vi "Set Duty Cycle.vi"   [LabVIEW 2011, in "LMH-LINX.lvlib"]
doc: "Set the duty cycle of the specified PWM channel. \n\nA duty cycle of 0 coresponds to 0% on\nA duty cycle of .33 coresponds to 33% on\nA duty cycle of 1 coresponds to 100% on\netc"
uses:
  LMH-LINX.lvlib
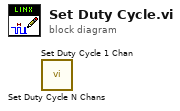
[diagram p0: block diagram]
diagram:
  n1 = call "Set Duty Cycle N Chans.vi"() -> ()  [unwired: 10 in, 2 out]
  n2 = call "Set Duty Cycle 1 Chan.vi"() -> ()  [unwired: 10 in, 2 out]
